vi "Read Gain Limits.vi"(8 "error in (no error)":errorcluster, 11 "APDClass in":refnum<class "APDClass.lvclass">) -> (0 "error out":errorcluster, 2 "GainLimits":cluster{"GainMin":dbl, "GainMax":dbl}, 3 "APDClass out":refnum<class "APDClass.lvclass">)   [LabVIEW 2019, in "APDClass.lvclass"]
uses:
  APDClass.lvclass
  APDClass.lvclass/APDClass.ctl
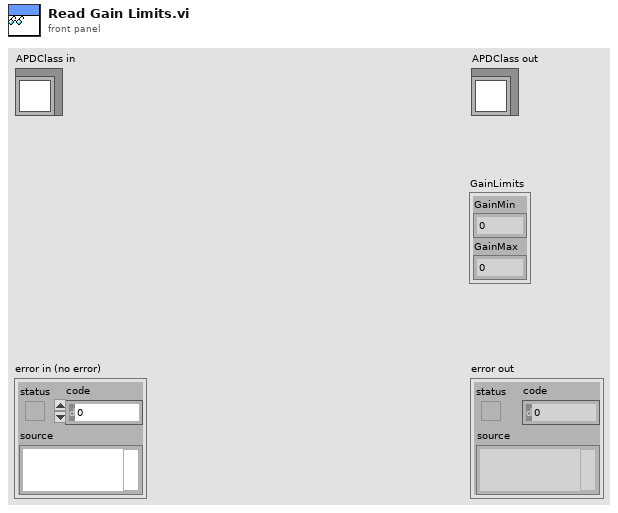
[diagram p1: front panel]
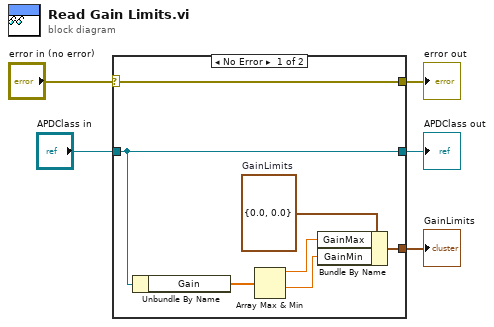
[diagram p0: block diagram]
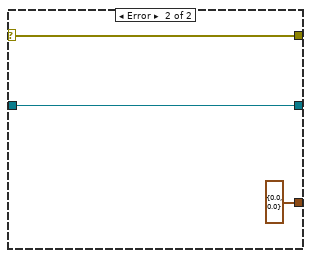
[diagram p2: hidden frame]
diagram:
  n1 = case shown="No Error" "error in (no error)" {
    selector: "error in (no error)" -> [w12 w14]
    tunnel: [w12 w14] -> w4
    tunnel: [w11 w15] -> w2
    tunnel: "APDClass in" -> [w11 w15]
    tunnel: [w6 cluster{"GainMin":dbl, "GainMax":dbl} {"GainMin"=0.0, "GainMax"=0.0} ("GainMinMax")] -> w1
    frame No Error {
      w9 = cluster{"GainMin":dbl, "GainMax":dbl} {"GainMin"=0.0, "GainMax"=0.0}  # GainLimits
      n2 = Unbundle By Name(w11) -> ("Gain"=w10:dbl[])
      n3 = Array Max & Min(array=w10) -> (max value=w7:dbl, min value=w8:dbl)  [unwired: 2 out]
      n4 = Bundle By Name(cluster=w9, "GainMax"=w7, "GainMin"=w8) -> (w6:cluster{"GainMin":dbl, "GainMax":dbl})
    }
    frame Error {
    }
  }
  "error out" <- w4
  "APDClass out" <- w2
  "GainLimits" <- w1
